vi "PNA_Delay.vi"(2 "error in (no error)":errorcluster, 3 "Delay (0 ns)":dbl, 4 "Channel (1)":i32=1, 5 "VISA resource name":refnum<visa-resource-name>) -> (0 "error out":errorcluster, 1 "VISA resource name out":refnum<visa-resource-name>)   [LabVIEW 2020]
uses:
  <instrlib>/Keysight PNA Series/Keysight PNA Series.lvlib
panel:
  out "resulting string":string
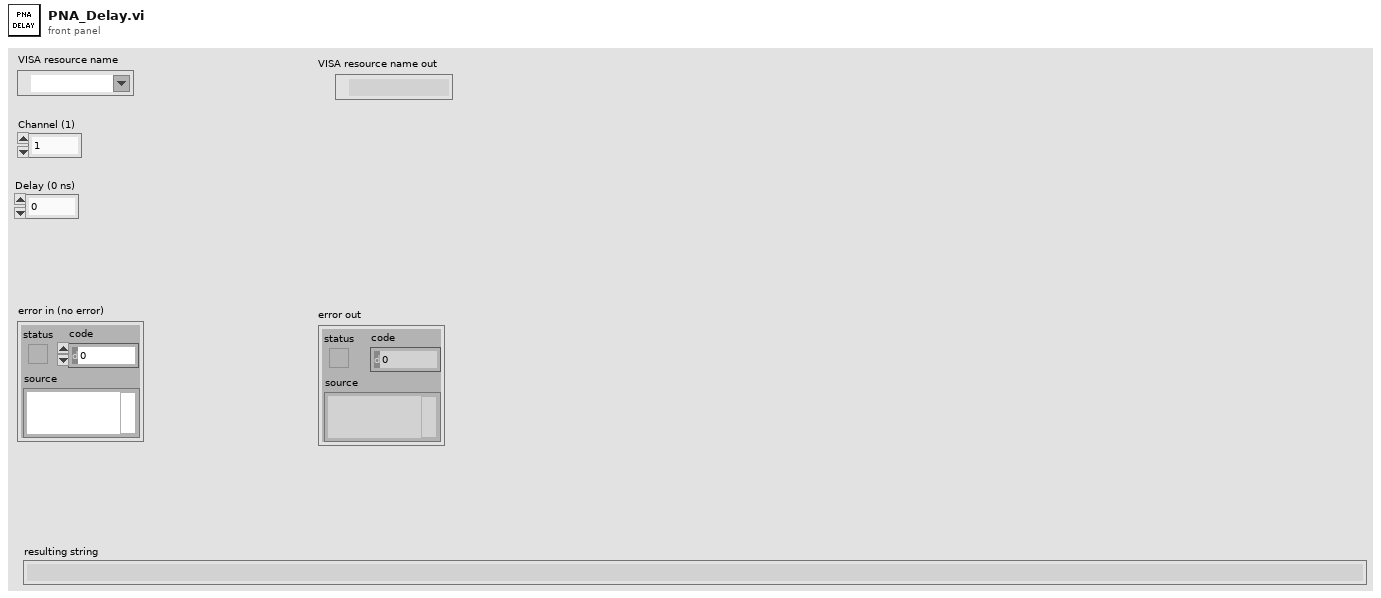
[diagram p1: front panel]
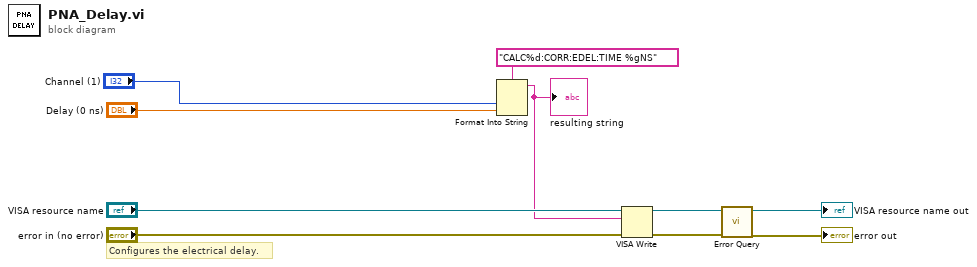
[diagram p0: block diagram]
diagram:
  # "Configures the electrical delay."
  n1 = Format Into String(format string="CALC%d:CORR:EDEL:TIME %gNS", "Channel (1)", "Delay (0 ns)") -> (resulting string=w1:string)  [unwired: 2 in, 1 out]
  "resulting string" <- w1
  n2 = VISA Write(VISA resource name="VISA resource name", write buffer=w1, error in (no error)="error in (no error)") -> (VISA resource name out=w5:refnum<visa-resource-name>, error out=w4:errorcluster)  [unwired: 1 out]
  n3 = call <instrlib>:"Error Query.vi"("error in (no error)"=w4, "VISA resource name"=w5) -> ("error out"=→"error out":errorcluster, "VISA resource name out"=→"VISA resource name out":refnum<visa-resource-name>)  [unwired: 6 in, 2 out]
